vi "SmartPowerGrid.vi"() -> ()   [LabVIEW 2018]
panel:
  in  "gsm(wifi) led count 3":i32
  out "?":bool
  out "?":bool
  out "?":bool
  out "?":bool
  in  "gsm(wifi) led count 2":i32
  out "?":bool
  out "?":bool
  out "?":bool
  out "?":bool
  out "?":bool
  out "?":bool
  out "?":bool
  out "?":bool
  in  "gsm(wifi) led count":i32
  out "Waveform Graph 3":dynamicdata(graph)
  out "Waveform Graph 2":dynamicdata(graph)
  out "Waveform Graph":dynamicdata(graph)
  out "control station":string
  in  "ip power t1 3":i32
  out "digital 3":bool
  in  "digitizer 3":dbl
  in  "milliseconds to wait 3":u32
  out "digital3":bool
  in  "power loss t1 3":dbl
  out "power loss detected 3":bool
  out "concatenated string t1 3":string
  out "op power t1 3":dbl
  in  "loop count 3":dbl
  in  "ip power t1 2":i32
  out "digital 2":bool
  in  "digitizer 2":dbl
  in  "milliseconds to wait 2":u32
  out "digital2":bool
  in  "power loss t1 2":dbl
  out "power loss detected 2":bool
  out "concatenated string t1 2":string
  out "op power t1 2":dbl
  in  "loop count 2":dbl
  out "concatenated string t1":string
  out "power loss detected":bool
  in  "power loss t1":dbl
  out "digital 1":bool
  in  "milliseconds to wait":u32
  in  "digitizer":dbl
  out "op power t1":dbl
  in  "ip  power t1":i32
  out "digital 0":bool
  in  "loop count":dbl
  # "transformer 1"
  # "transformer 2"
  # "transformer 3"
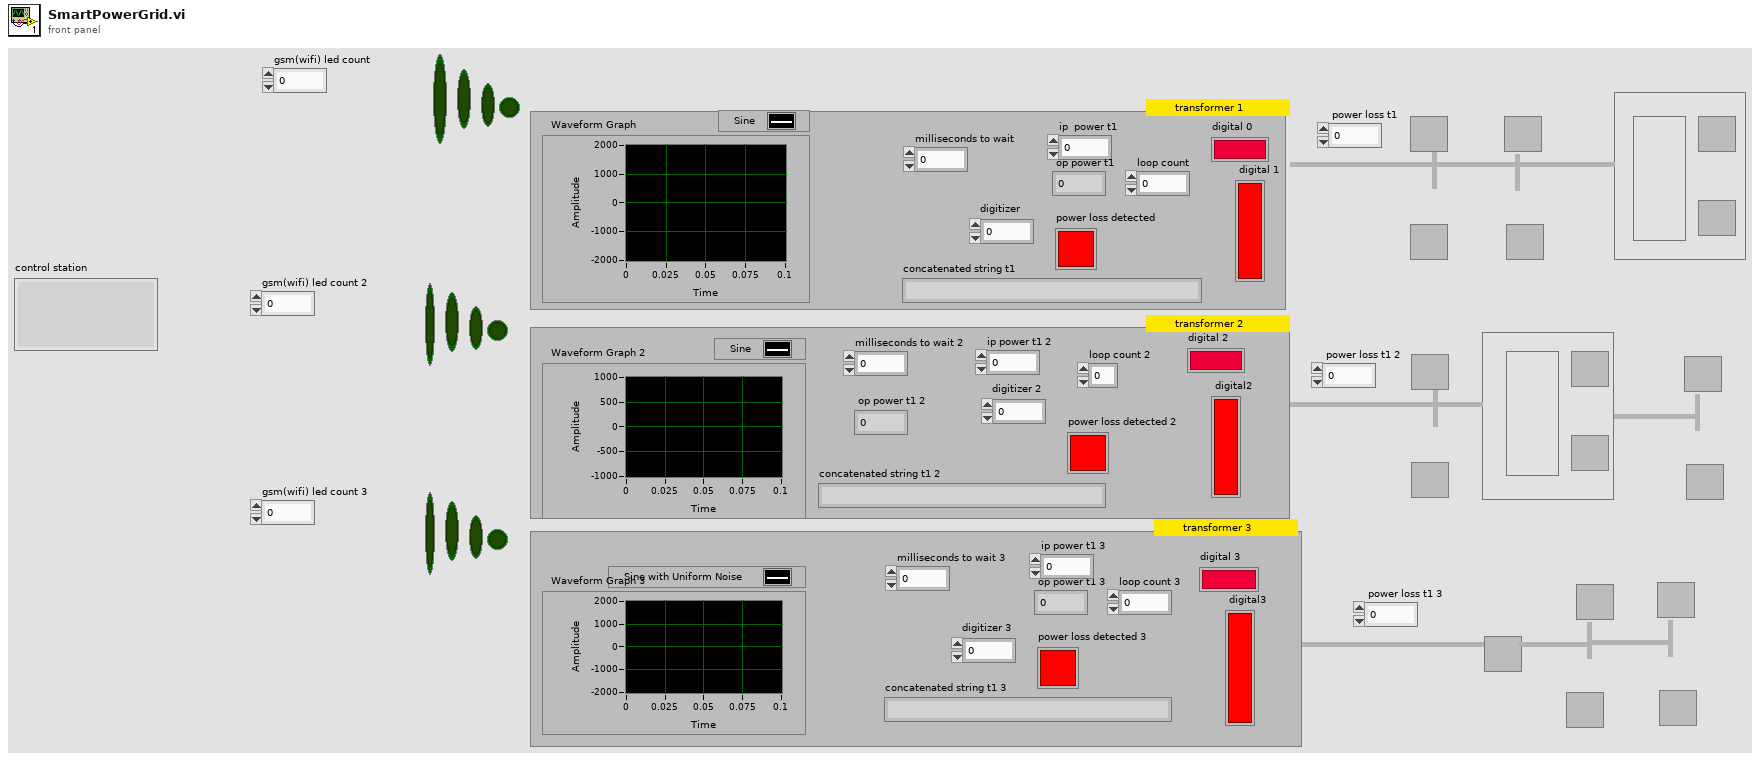
[diagram p1: front panel]
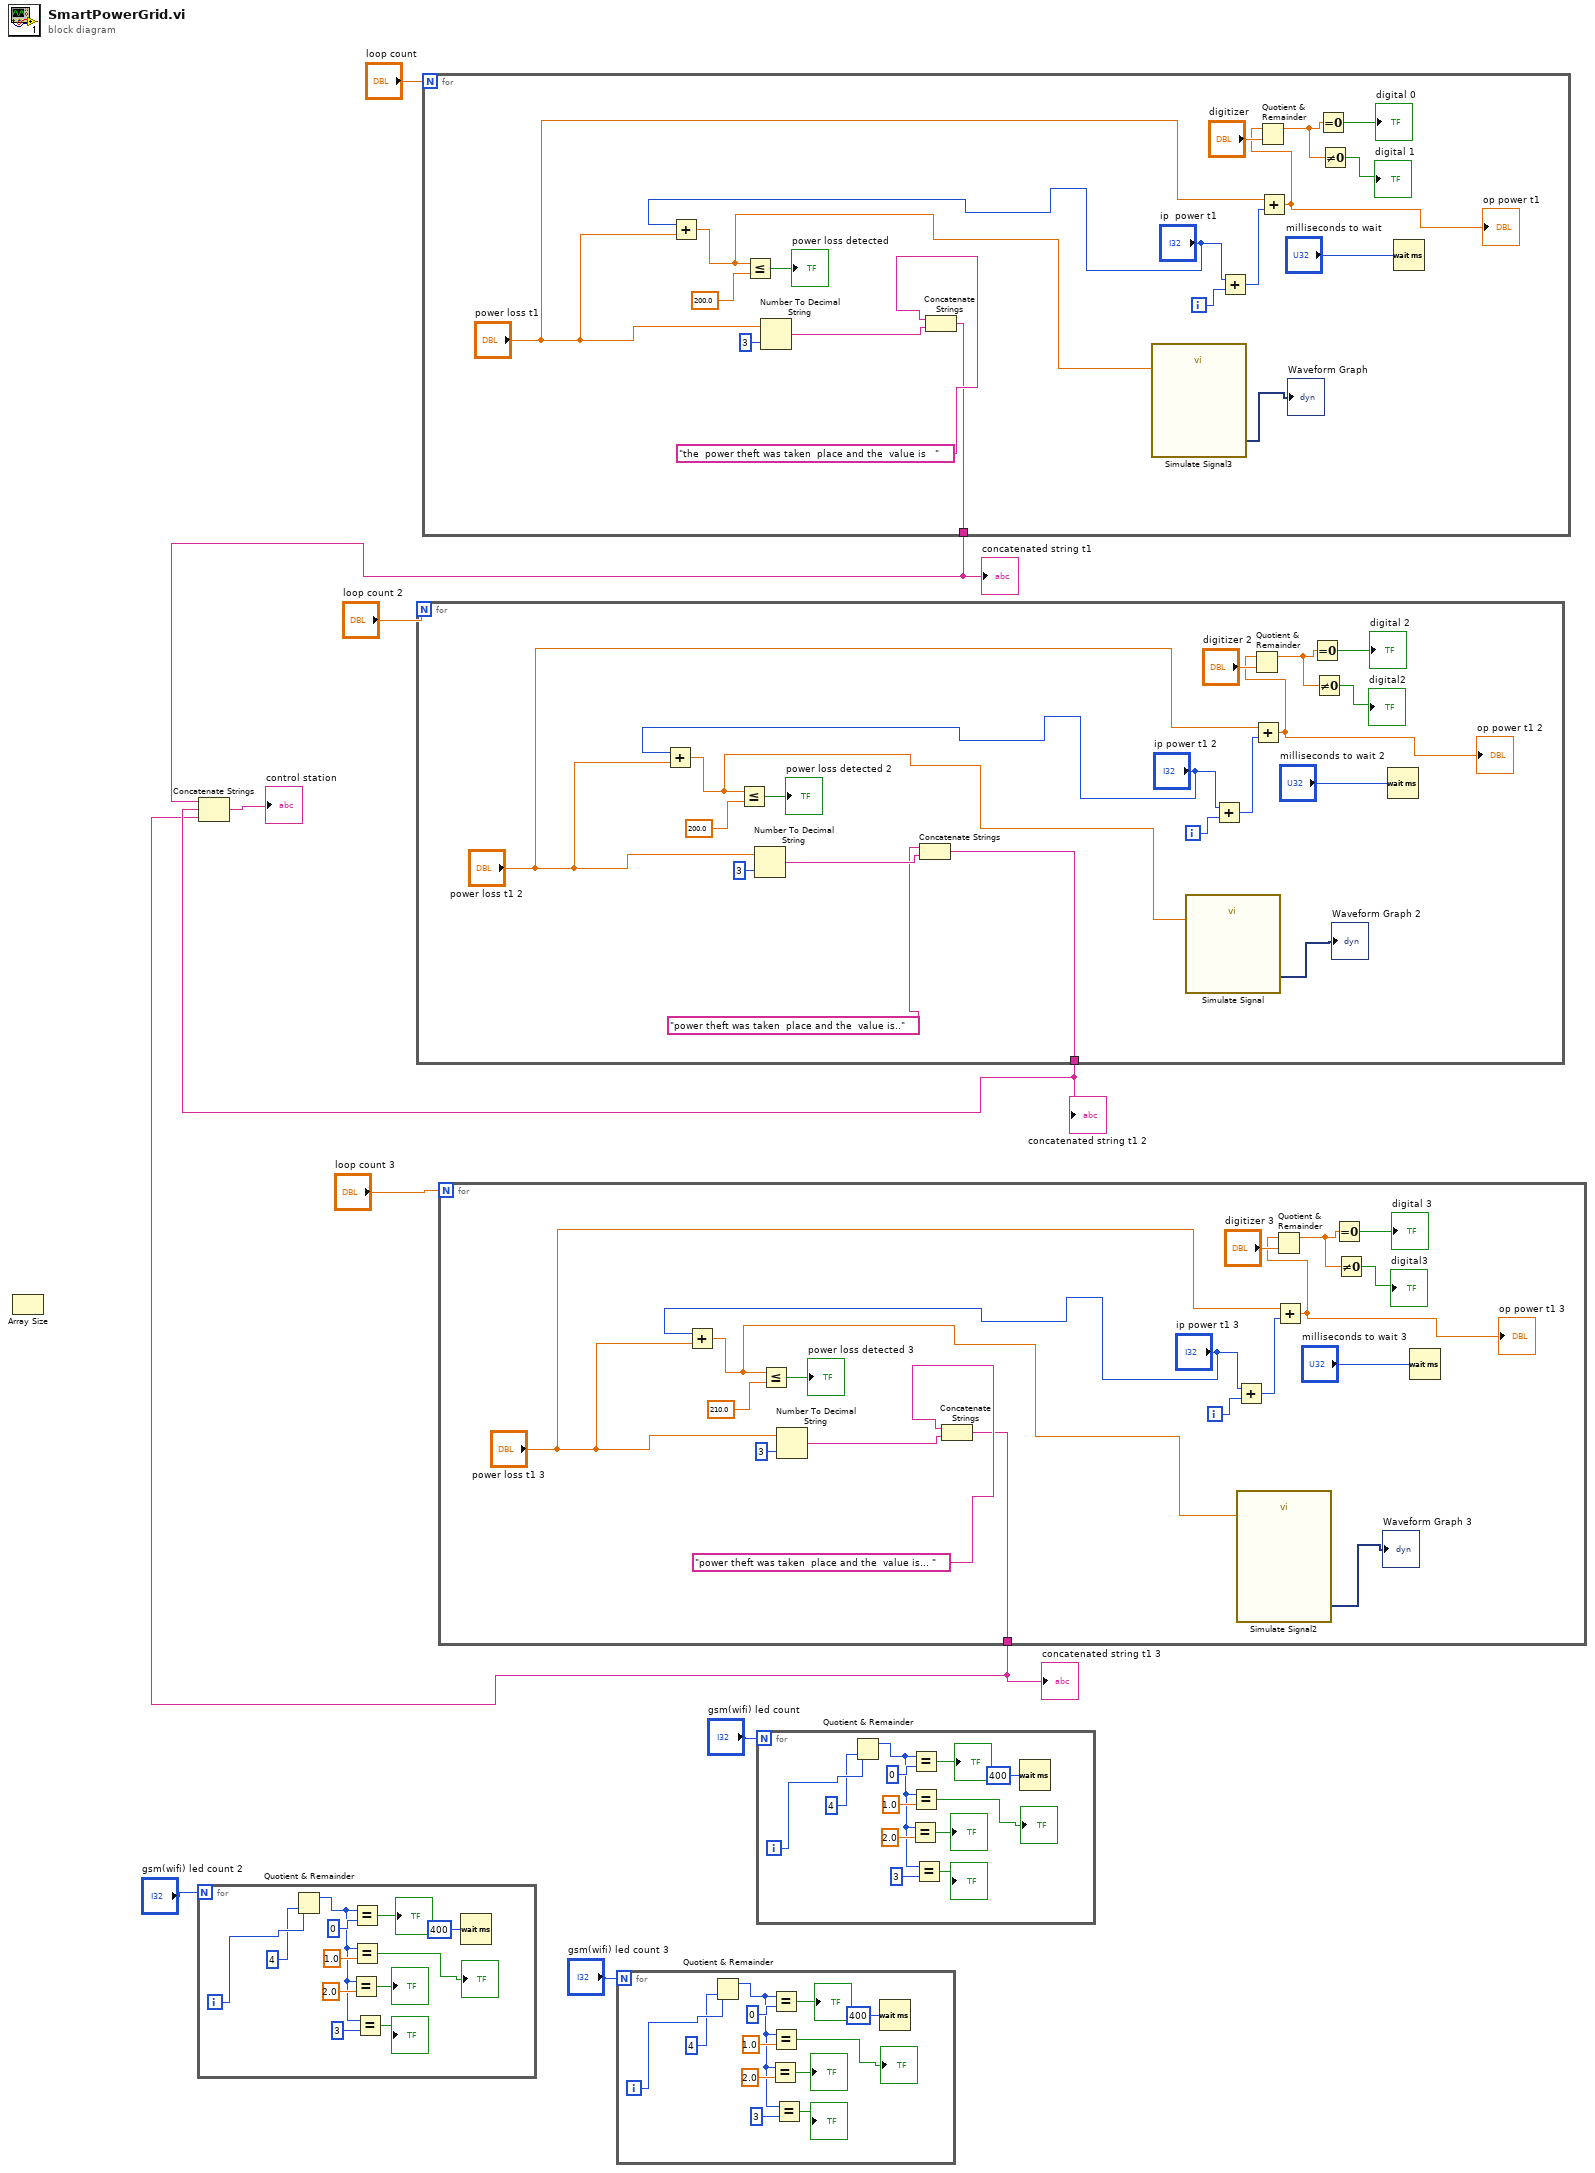
[diagram p0: block diagram]
diagram:
  n1 = Array Size() -> ()  [unwired: 1 in, 1 out]
  n2 = for {
    N: "gsm(wifi) led count 2" -> [_]
    i -> [w22]
    n3 = Quotient & Remainder(x=w22, y=4) -> (x-y*floor(x/y)=w13:i32)  [unwired: 1 out]
    n4 = Equal?(x=w13, y=2.0) -> (x = y?=→"?":bool)
    n5 = Equal?(x=w13, y=0) -> (x = y?=→"?":bool)
    n6 = Equal?(x=w13, y=1.0) -> (x = y?=→"?":bool)
    n7 = Equal?(x=w13, y=3) -> (x = y?=→"?":bool)
    n8 = Wait (ms)(milliseconds to wait=u32 400) -> ()  [unwired: 1 out]
  }
  n9 = for {
    N: "loop count 2" -> [_]
    tunnel: [w25] -> w6
    i -> [w40]
    n10 = Add(x="ip power t1 2", y="power loss t1 2") -> (x+y=w23:dbl)
    n11 = Less Or Equal?(x=w23, y=200.0) -> (x <= y?=→"power loss detected 2":bool)
    n12 = Number To Decimal String(number="power loss t1 2", width (-)=i16 3) -> (decimal integer string=w30:string)
    n13 = Concatenate Strings("power theft was taken  place and the  value is..", w30) -> (w25:string)
    n14 = call "Simulate Signal"("Amplitude"=w23) -> ("Sine"=→"Waveform Graph 2":dynamicdata)  [unwired: 13 in, 1 out]
    n15 = Add(x="ip power t1 2", y=w40) -> (x+y=w39:i32)
    n16 = Add(x="power loss t1 2", y=w39) -> (x+y=w27:dbl)
    "op power t1 2" <- w27
    n17 = Quotient & Remainder(x=w27, y="digitizer 2") -> (x-y*floor(x/y)=w35:dbl)  [unwired: 1 out]
    n18 = Equal To 0?(x=w35) -> (x = 0?=→"digital 2":bool)
    n19 = Not Equal To 0?(x=w35) -> (x != 0?=→"digital2":bool)
    n20 = Wait (ms)(milliseconds to wait="milliseconds to wait 2") -> ()  [unwired: 1 out]
  }
  "concatenated string t1 2" <- w6
  n21 = for {
    N: "loop count" -> [_]
    tunnel: [w43] -> w7
    i -> [w58]
    n22 = Add(x="ip  power t1", y="power loss t1") -> (x+y=w41:dbl)
    n23 = Less Or Equal?(x=w41, y=200.0) -> (x <= y?=→"power loss detected":bool)
    n24 = Number To Decimal String(number="power loss t1", width (-)=i16 3) -> (decimal integer string=w47:string)
    n25 = Concatenate Strings("the  power theft was taken  place and the  value is   ", w47) -> (w43:string)
    n26 = call "Simulate Signal3"("Amplitude"=w41) -> ("Sine"=→"Waveform Graph":dynamicdata)  [unwired: 13 in, 1 out]
    n27 = Add(x="ip  power t1", y=w58) -> (x+y=w57:i32)
    n28 = Add(x="power loss t1", y=w57) -> (x+y=w44:dbl)
    "op power t1" <- w44
    n29 = Quotient & Remainder(x=w44, y="digitizer") -> (x-y*floor(x/y)=w53:dbl)  [unwired: 1 out]
    n30 = Equal To 0?(x=w53) -> (x = 0?=→"digital 0":bool)
    n31 = Not Equal To 0?(x=w53) -> (x != 0?=→"digital 1":bool)
    n32 = Wait (ms)(milliseconds to wait="milliseconds to wait") -> ()  [unwired: 1 out]
  }
  "concatenated string t1" <- w7
  n33 = for {
    N: "loop count 3" -> [_]
    tunnel: [w61] -> w5
    i -> [w76]
    n34 = Add(x="ip power t1 3", y="power loss t1 3") -> (x+y=w59:dbl)
    n35 = Less Or Equal?(x=w59, y=210.0) -> (x <= y?=→"power loss detected 3":bool)
    n36 = Number To Decimal String(number="power loss t1 3", width (-)=i16 3) -> (decimal integer string=w65:string)
    n37 = Concatenate Strings("power theft was taken  place and the  value is... ", w65) -> (w61:string)
    n38 = Add(x="ip power t1 3", y=w76) -> (x+y=w75:i32)
    n39 = call "Simulate Signal2"("Amplitude"=w59) -> ("Sine with Uniform Noise"=→"Waveform Graph 3":dynamicdata)  [unwired: 13 in, 1 out]
    n40 = Add(x="power loss t1 3", y=w75) -> (x+y=w62:dbl)
    "op power t1 3" <- w62
    n41 = Quotient & Remainder(x=w62, y="digitizer 3") -> (x-y*floor(x/y)=w71:dbl)  [unwired: 1 out]
    n42 = Equal To 0?(x=w71) -> (x = 0?=→"digital 3":bool)
    n43 = Not Equal To 0?(x=w71) -> (x != 0?=→"digital3":bool)
    n44 = Wait (ms)(milliseconds to wait="milliseconds to wait 3") -> ()  [unwired: 1 out]
  }
  "concatenated string t1 3" <- w5
  n45 = Concatenate Strings(w7, w6, w5) -> (→"control station":string)
  n46 = for {
    N: "gsm(wifi) led count 3" -> [_]
    i -> [w88]
    n47 = Quotient & Remainder(x=w88, y=4) -> (x-y*floor(x/y)=w79:i32)  [unwired: 1 out]
    n48 = Equal?(x=w79, y=2.0) -> (x = y?=→"?":bool)
    n49 = Equal?(x=w79, y=0) -> (x = y?=→"?":bool)
    n50 = Equal?(x=w79, y=1.0) -> (x = y?=→"?":bool)
    n51 = Equal?(x=w79, y=3) -> (x = y?=→"?":bool)
    n52 = Wait (ms)(milliseconds to wait=u32 400) -> ()  [unwired: 1 out]
  }
  n53 = for {
    N: "gsm(wifi) led count" -> [_]
    i -> [w100]
    n54 = Quotient & Remainder(x=w100, y=4) -> (x-y*floor(x/y)=w91:i32)  [unwired: 1 out]
    n55 = Equal?(x=w91, y=2.0) -> (x = y?=→"?":bool)
    n56 = Equal?(x=w91, y=0) -> (x = y?=→"?":bool)
    n57 = Equal?(x=w91, y=1.0) -> (x = y?=→"?":bool)
    n58 = Equal?(x=w91, y=3) -> (x = y?=→"?":bool)
    n59 = Wait (ms)(milliseconds to wait=u32 400) -> ()  [unwired: 1 out]
  }
